vi "Initial.vi"(8 "error in (no error)":errorcluster, 11 "DMC_1000B in":refnum<class "DMC_1000B.lvclass">) -> (0 "error out":errorcluster, 3 "DMC_1000B out":refnum<class "DMC_1000B.lvclass">)   [LabVIEW 2019, in "DMC_1000B.lvclass"]
uses:
  DMC_1000B.lvclass
  IO Folder/IO_Class/IOCard.lvclass
  LLB/Commonly VI.lvlib
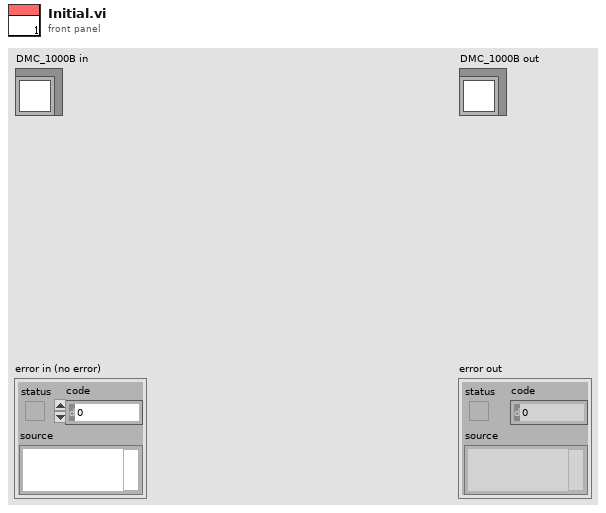
[diagram p1: front panel]
types:
  T1 = cluster{"Card":i32, "Connect":bool, "Handler":i32}[]
  T2 = cluster{"Card":i32, "Connect":bool, "Handler":i32}
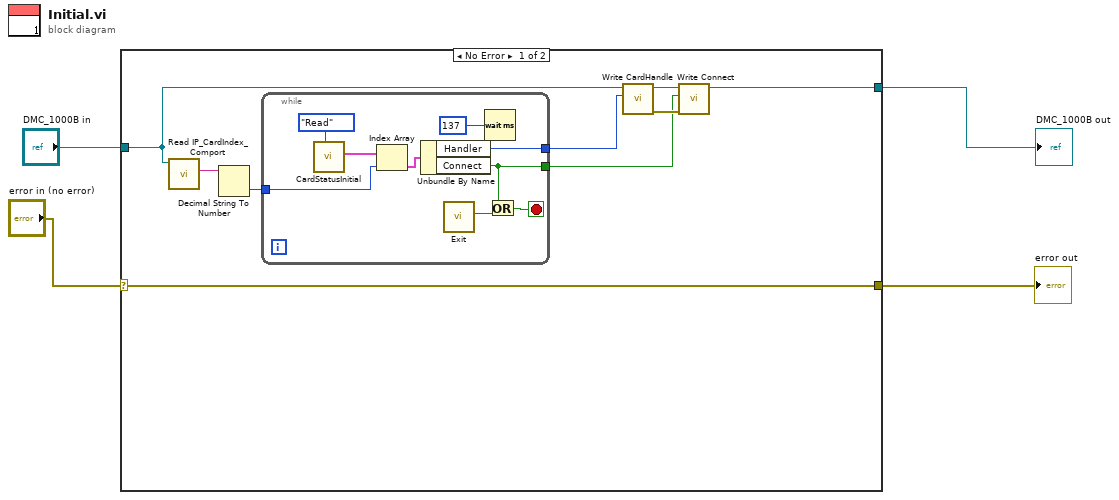
[diagram p0: block diagram]
diagram:
  n1 = case shown="No Error" "error in (no error)" {
    selector: "error in (no error)" -> [w11 w23]
    tunnel: "DMC_1000B in" -> [w10 w24]
    tunnel: [w6 w24] -> w2
    tunnel: [w11 w23] -> w1
    frame No Error {
      n2 = call-dynamic "Read IP_CardIndex_Comport.vi"("AxisCard in"=w10) -> ("IP/CardIndex/Comport"=w13:string)  [unwired: 8 in, 2 out]
      n3 = Decimal String To Number(string=w13) -> (number=w12:i32)  [unwired: 2 in, 1 out]
      n4 = while {
        tunnel: w12 -> [w16]
        tunnel: [w15] -> w9
        tunnel: [w14] -> w5
        stop <- w17 stop-if-true
        n5 = call "CardStatusInitial.vi"("Action"=enum16{"Initial", "Write", "Read", "Release"}."Read") -> ("CardStatus"=w21:T1)  [unwired: 10 in]
        n6 = Index Array(array=w21, index=w16) -> (element=w20:T2)
        n7 = Unbundle By Name(w20) -> ("Handler"=w15:i32, "Connect"=w14:bool)
        n8 = call "Exit.vi"() -> ("ExitOut"=w18:bool)  [unwired: 11 in]
        n9 = Wait (ms)(milliseconds to wait=u32 137) -> ()  [unwired: 1 out]
        n10 = Or(x=w14, y=w18) -> (x .or. y?=w17:bool)
      }
      n11 = call-dynamic "Write CardHandle.vi"("CardHandle"=w9, "AxisCard in"=w10) -> ("error out"=w8:errorcluster, "AxisCard out"=w7:refnum<class "DMC_1000B.lvclass">)  [unwired: 8 in]
      n12 = call-dynamic "Write Connect.vi"("error in (no error)"=w8, "Connect"=w5, "AxisCard in"=w7) -> ("AxisCard out"=w6:refnum<class "DMC_1000B.lvclass">)  [unwired: 7 in, 1 out]
    }
    frame Error {
    }
  }
  "error out" <- w1
  "DMC_1000B out" <- w2
